vi "sub_HandleOutput.vi"(7 "Output file text box":refnum<k7>(container), 8 "error in (no error)":errorcluster, 10 "Dynamic data":T1, 11 "Input parameters":T2={"Measurement type"=enum."Test", "Sensor type"=enum."HPK_8in_256", "Identifier"="test.txt", "Open after execution?"=FALSE, "Plot after execution?"=FALSE, "Display channel"=0, "Voltage Delay (s)"=0.5, "Switch Delay (s)"=0.01, "VISA resource name source"="", "VISA resource name DMM"="", "VISA resource name LCR"="", "Compliance  Level (uA)"=10.0, "Voltage Limit (V)"=1000.0, "Data storage location"="", "Scan voltages"="", "Use source as DMM?"=FALSE, "Single channel?"=FALSE, "LCR signal frequenzy (Hz)"=10.0, "DMM device"=enum."Keithley2001", "Sampling number"=1} {"Voltage Limit (V)" format="%#_13g"; "Voltage Delay (s)" format="%#_13g"; "Switch Delay (s)" format="%#_13g"}) -> (0 "error out":errorcluster, 2 "Dynamic data":T1, 3 "Input parameters":T2={"Measurement type"=enum."Test", "Sensor type"=enum."HPK_8in_256", "Identifier"="test.txt", "Open after execution?"=FALSE, "Plot after execution?"=FALSE, "Display channel"=0, "Voltage Delay (s)"=0.5, "Switch Delay (s)"=0.01, "VISA resource name source"="", "VISA resource name DMM"="", "VISA resource name LCR"="", "Compliance  Level (uA)"=10.0, "Voltage Limit (V)"=1000.0, "Data storage location"="", "Scan voltages"="", "Use source as DMM?"=FALSE, "Single channel?"=FALSE, "LCR signal frequenzy (Hz)"=10.0, "DMM device"=enum."Keithley2001", "Sampling number"=1} {"Voltage Limit (V)" format="%#_13g"; "Voltage Delay (s)" format="%#_13g"; "Switch Delay (s)" format="%#_13g"})   [LabVIEW 2016]
uses:
  Input_parameters.ctl
  Dynamic_data.ctl
  <vilib>/Utility/file.llb/Write Delimited Spreadsheet (string).vi
panel:
  out "standard error":string
  out "standard output":string
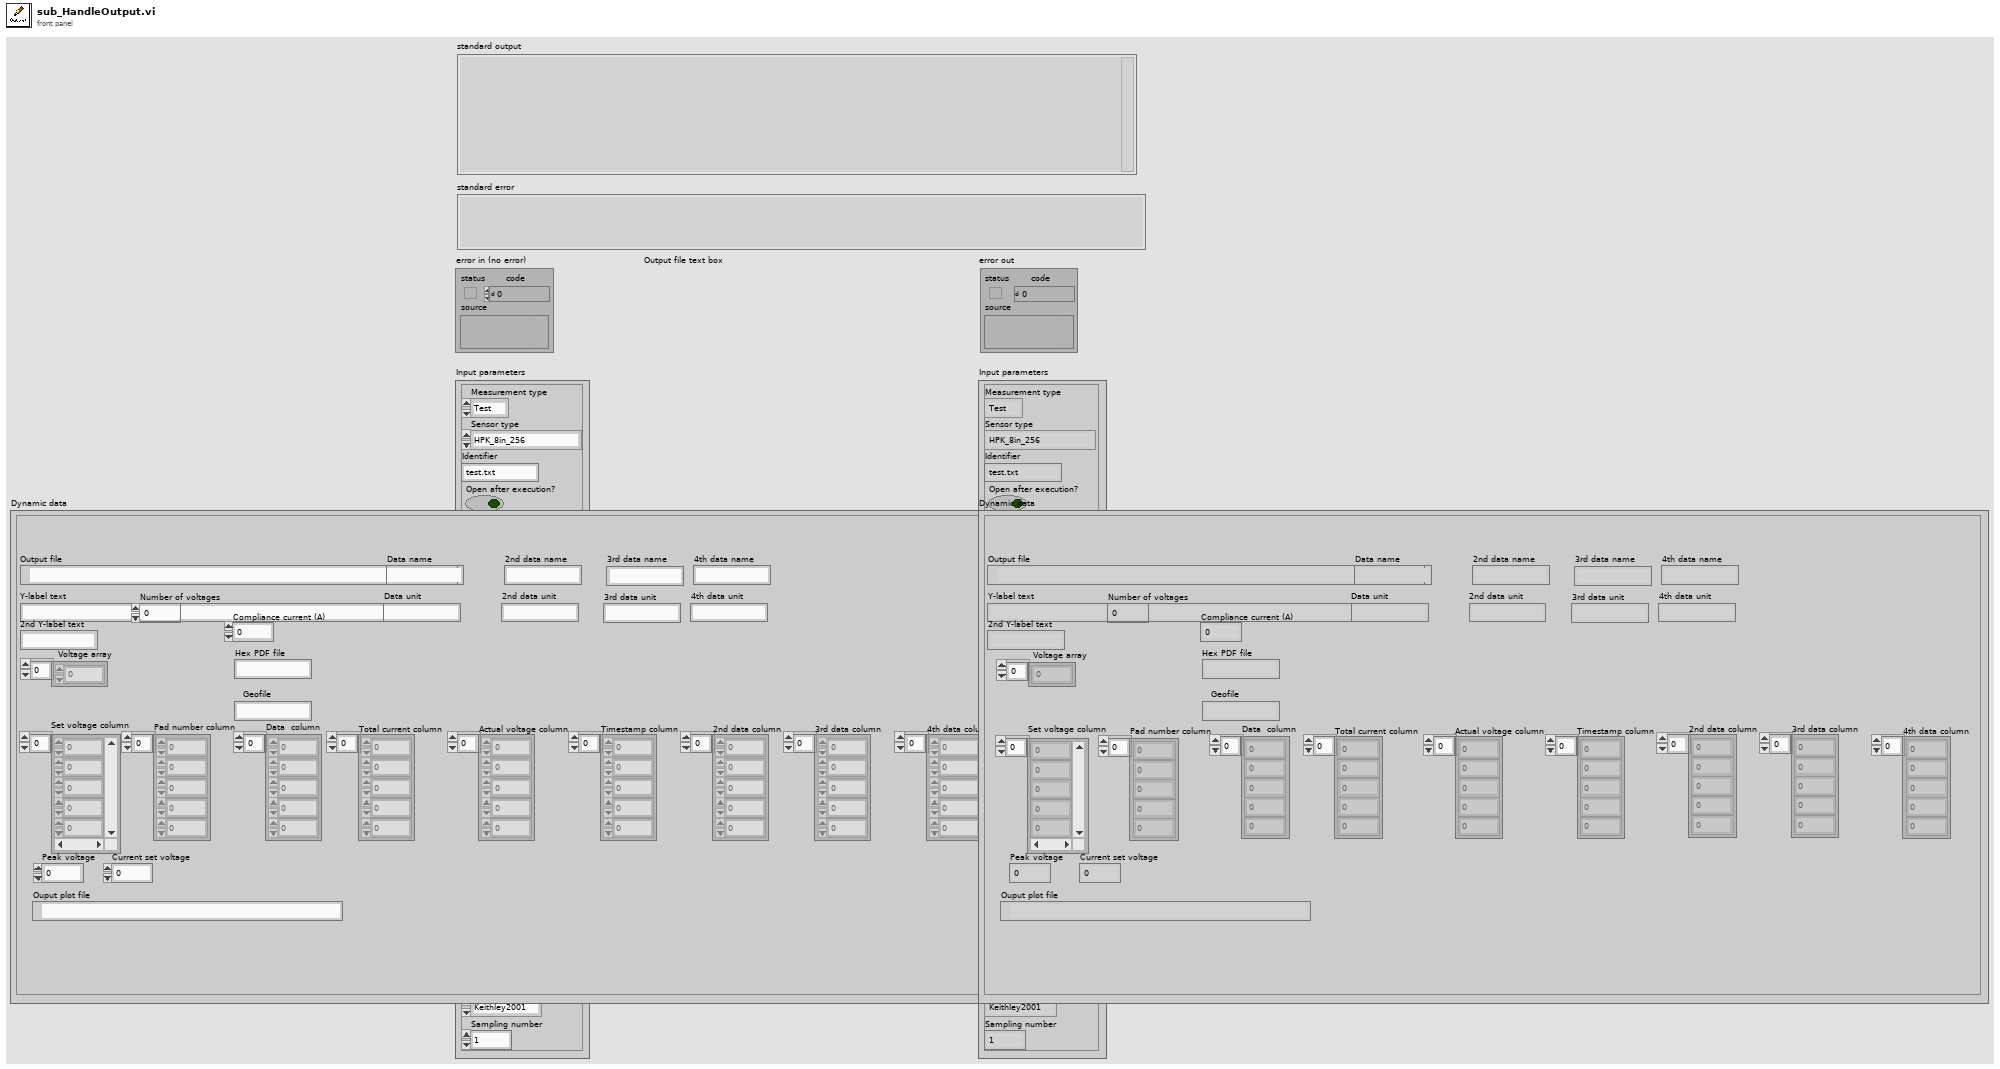
[diagram p1: front panel]
types:
  T1 = typedef "Dynamic_data.ctl" = cluster{"Output file":path, "Y-label text":string, "Current set voltage":dbl, "Set voltage column":dbl[], "Pad number column":dbl[], "Data  column":dbl[], "Number of voltages":i32, "Compliance current (A)":dbl, "Geofile":string, "Peak voltage":dbl, "Hex PDF file":string, "Voltage array":dbl[], "Total current column":dbl[], "Timestamp column":dbl[], "Data name":string, "Data unit":string, "2nd data column":dbl[], "2nd data name":string, "2nd data unit":string, "3rd data column":dbl[], "4th data column":dbl[], "3rd data name":string, "3rd data unit":string, "4th data name":string, "4th data unit":string, "Actual voltage column":dbl[], "2nd Y-label text":string, "Ouput plot file":path}
  T2 = typedef "Input_parameters.ctl" = cluster{"Measurement type":enum16{"IV", "CV", "Test"}, "Sensor type":enum16{"HPK_6in_135", "HPK_8in_256", "INF_8in_256", "Diode", "HPK_6in_256"}, "Identifier":string, "Open after execution?":bool, "Plot after execution?":bool, "Display channel":i32, "Voltage Delay (s)":dbl, "Switch Delay (s)":dbl, "VISA resource name source":refnum<visa-resource-name>, "VISA resource name DMM":refnum<visa-resource-name>, "VISA resource name LCR":refnum<visa-resource-name>, "Compliance  Level (uA)":dbl, "Voltage Limit (V)":dbl, "Data storage location":string, "Scan voltages":string, "Use source as DMM?":bool, "Single channel?":bool, "LCR signal frequenzy (Hz)":dbl, "DMM device":enum16{"Keithley2001", "Keithley2450", "Keithley2410"}, "Sampling number":i32}
  T3 = enum16{"HPK_6in_135", "HPK_8in_256", "INF_8in_256", "Diode", "HPK_6in_256"}
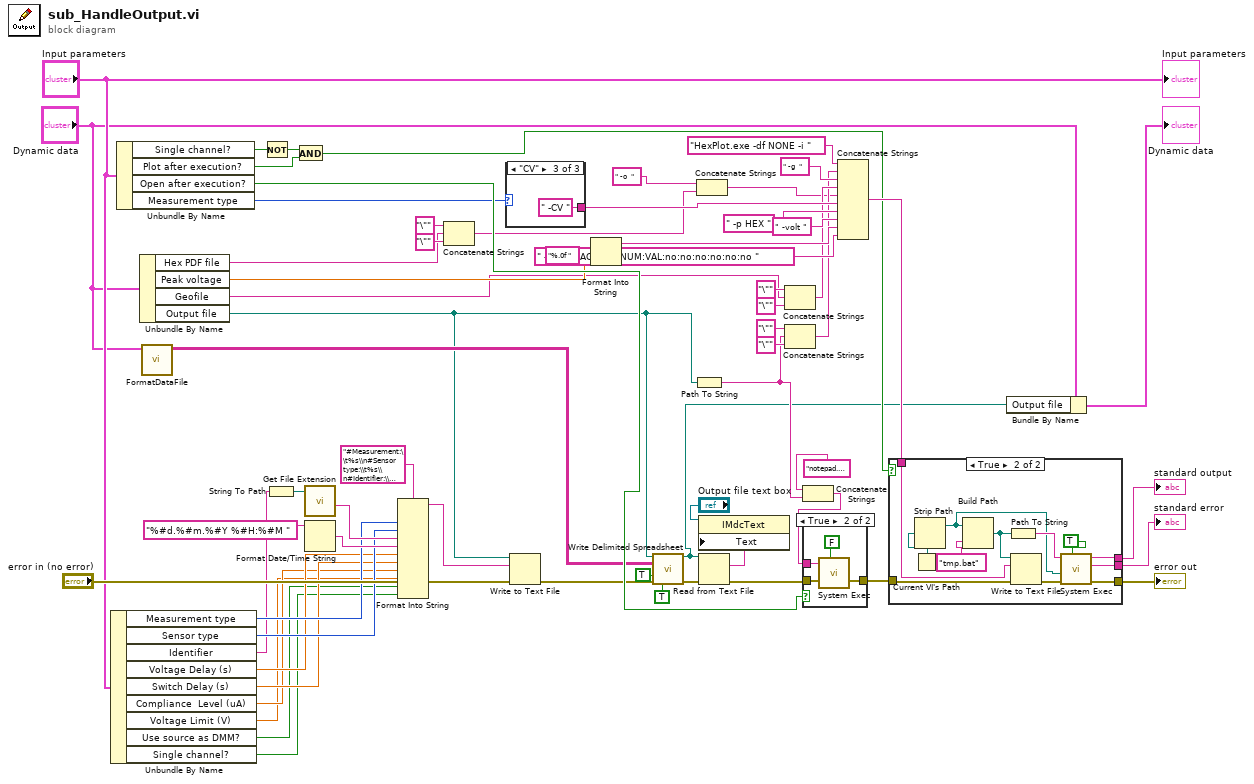
[diagram p0: block diagram]
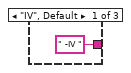
[diagram p2: hidden frame]
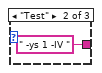
[diagram p3: hidden frame]
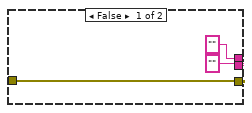
[diagram p4: hidden frame]
diagram:
  n1 = Unbundle By Name("Input parameters") -> ("Measurement type"=w12:enum16{"IV", "CV", "Test"}, "Sensor type"=w11:T3, "Identifier"=w10:string, "Voltage Delay (s)"=w9:dbl, "Switch Delay (s)"=w8:dbl, "Compliance  Level (uA)"=w7:dbl, "Voltage Limit (V)"=w6:dbl, "Use source as DMM?"=w4:bool, "Single channel?"=w5:bool)
  n2 = Unbundle By Name("Input parameters") -> ("Single channel?"=w14:bool, "Plot after execution?"=w19:bool, "Open after execution?"=w62:bool, "Measurement type"=w25:enum16{"IV", "CV", "Test"})
  n3 = Unbundle By Name("Dynamic data") -> ("Hex PDF file"=w38:string, "Peak voltage"=w55:dbl, "Geofile"=w42:string, "Output file"=w1:path)
  n4 = call "FormatDataFile.vi"("Dynamic data"="Dynamic data") -> ("appended array"=w3:string[][])  [unwired: 10 in]
  n5 = Not(x=w14) -> (.not. x?=w18:bool)
  n6 = String To Path(string=w10) -> (path=w29:path)
  n7 = And(x=w18, y=w19) -> (x .and. y?=w24:bool)
  n8 = call <vilib>:"Get File Extension.vi"("file"=w29) -> ("filename without extension"=w28:string)  [unwired: 6 in, 4 out]
  n9 = Format Date/Time String(time format string (%c)="%#d.%#m.%#Y %#H:%#M ") -> (date/time string=w16:string)  [unwired: 2 in]
  n10 = Format Into String(format string="#Measurement:\\t%s\\n#Sensor type:\\t%s\\n#Identifier:\\t%s\\n#Timestamp:\\t%s\\n#Voltage delay:\\t%.1f s\\n#Switch delay:\\t%.1f s\\n#Compliance level:\\t%.2f uA\\n#Voltage limit:\\t%.1f V\\n#Source as DMM:\\t%d\\n#Single channel:\\t%d\\n\\n", w12, w11, w28, w16, w9, w8, w7, w6, w4, w5) -> (resulting string=w30:string)  [unwired: 2 in, 1 out]
  n11 = Concatenate Strings("\"" ("string"), w38, "\"" ("string")) -> (w39:string)
  n12 = case shown="\"CV\"" w25 {
    tunnel: [" -IV " ("string") " -ys 1 -IV " ("string") " -CV " ("string")] -> w58
    frame "IV", Default {
    }
    frame "Test" {
    }
    frame "CV" {
    }
  }
  n13 = Write to Text File(file (use dialog)=w1, text=w30, error in="error in (no error)") -> (error out=w32:errorcluster)  [unwired: 1 in, 2 out]
  n14 = Format Into String(format string="%.0f ", w55) -> (resulting string=w53:string)  [unwired: 2 in, 1 out]
  n15 = call-poly <vilib>:"Write Delimited Spreadsheet.vi"("file path (dialog if empty)"=w1, "2D data"=w3, "append to file? (new file:F)"=TRUE, "error in (no error)"=w32, "transpose? (no:F)"=TRUE) -> ("new file path (Not A Path if cancelled)"=w20:path, "error out"=w22:errorcluster)  [unwired: 9 in]
  n16 = Path To String(path=w1) -> (string=w23:string)
  n17 = Concatenate Strings(" -o  " ("string"), w39) -> (w44:string)
  n18 = Read from Text File(file (use dialog)=w20, error in=w22) -> (text=w34:string, error out=w21:errorcluster)  [unwired: 2 in, 2 out]
  n19 = property class="IMdcText"(reference="Output file text box", "Text"=w34) -> ()  [unwired: 1 in, 2 out]
  n20 = Concatenate Strings("\"" ("string"), w42, "\"" ("string")) -> (w49:string)
  n21 = Concatenate Strings("\"" ("string"), w23, "\"" ("string")) -> (w46:string)
  n22 = Concatenate Strings("notepad.exe " ("string"), w23) -> (w63:string)
  n23 = case shown="True" w62 {
    tunnel: w63 -> [_ w73]
    tunnel: w21 -> [w69 w72]
    tunnel: [w69 w71] -> w26
    frame False {
    }
    frame True {
      n24 = call <vilib>:"System Exec.vi"("wait until completion? (T)"=FALSE, "error in (no error)"=w72, "command line"=w73) -> ("error out"=w71:errorcluster)  [unwired: 5 in, 3 out]
    }
  }
  n25 = Concatenate Strings("HexPlot.exe -df NONE -i " ("string"), w46, " -g  " ("string"), w49, w44, w58, " -p HEX " ("string"), " -volt " ("string"), w53, " -if VOLTAGE:PADNUM:VAL:no:no:no:no:no:no " ("string")) -> (w27:string)
  n26 = case shown="True" w24 {
    tunnel: [w76 w88] -> w45
    tunnel: w26 -> [w76 w80]
    tunnel: ["" ("standard output") w86] -> w37
    tunnel: ["" ("standard error") w85] -> w36
    tunnel: w27 -> [_ w81]
    frame False {
    }
    frame True {
      n27 = Current VI's Path() -> (path=w82:path)
      n28 = Strip Path(path=w82) -> (stripped path=w78:path)  [unwired: 1 out]
      n29 = Build Path(base path=w78, name or relative path="tmp.bat") -> (appended path=w84:path)
      n30 = Path To String(path=w84) -> (string=w79:string)
      n31 = Write to Text File(file (use dialog)=w84, text=w81, error in=w80) -> (error out=w77:errorcluster)  [unwired: 1 in, 2 out]
      n32 = call <vilib>:"System Exec.vi"("wait until completion? (T)"=TRUE, "error in (no error)"=w77, "working directory"=w78, "command line"=w79) -> ("error out"=w88:errorcluster, "standard error"=w85:string, "standard output"=w86:string)  [unwired: 4 in, 1 out]
    }
  }
  "error out" <- w45
  "standard output" <- w37
  "standard error" <- w36
  n33 = Bundle By Name(cluster="Dynamic data", "Output file"=w20) -> (→"Dynamic data":T1)
  "Input parameters" <- "Input parameters"
